vi "NodeFactory.vi"(8 "error in":errorcluster, 11 "reference":refnum<vi>) -> (0 "error out":errorcluster, 3 "Node out":refnum<class "Node.lvclass">)   [LabVIEW 2014, in "Raspberry Pi Compatible Compiler for LabVIEW.lvlib" / "Node.lvclass"]
uses:
  Node.lvclass
  Function/Function.lvclass
  Structure/Structure.lvclass
  GrowableFunction/GrowableFunction.lvclass
  SubVI/SubVI.lvclass
  Local/Local.lvclass
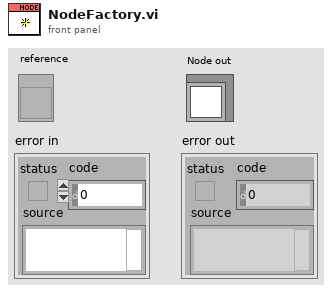
[diagram p1: front panel]
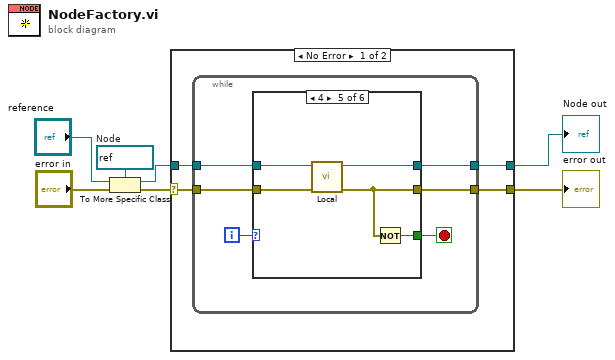
[diagram p0: block diagram]
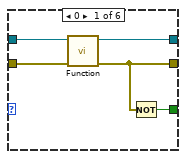
[diagram p2: hidden frame]
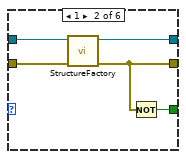
[diagram p3: hidden frame]
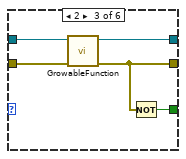
[diagram p4: hidden frame]
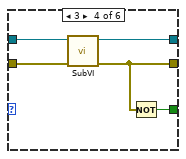
[diagram p5: hidden frame]
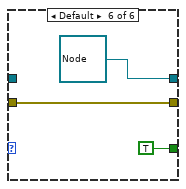
[diagram p6: hidden frame]
diagram:
  w5 = refnum<vi> refnum  # Node
  n1 = To More Specific Class(target class=w5, reference="reference", error in="error in") -> (specific class reference=w2:refnum<vi>, error out=w3:errorcluster)
  n2 = case shown="No Error" w3 {
    selector: w3 -> [w11 w46]
    tunnel: [w9 _] -> w7
    tunnel: [w8 w46] -> w6
    tunnel: w2 -> [w10 _]
    frame No Error {
      n3 = while {
        tunnel: w11 -> [w16]
        tunnel: [w15] -> w8
        tunnel: [w14] -> w9
        tunnel: w10 -> [w12]
        i -> [w17]
        stop <- w13 stop-if-true
        n4 = case shown="4" w17 {
          tunnel: w16 -> [w22 w27 w32 w37 w42 w44]
          tunnel: [w19 w24 w29 w34 w39 w44] -> w15
          tunnel: [w21 w26 w31 w36 w41 refnum<class "Node.lvclass"> refnum ("Node out")] -> w14
          tunnel: [w20 w25 w30 w35 w40 TRUE] -> w13
          tunnel: w12 -> [w18 w23 w28 w33 w38 _]
          frame 0 {
            n5 = call "Function.vi"("error in"=w22, "reference"=w18) -> ("error out"=w19:errorcluster, "Function out"=w21:refnum<class "Function.lvclass">)  [unwired: 8 in]
            n6 = Not(x=w19) -> (.not. x?=w20:bool)
          }
          frame 1 {
            n7 = call "StructureFactory.vi"("error in"=w27, "reference"=w23) -> ("error out"=w24:errorcluster, "structure out"=w26:refnum<class "Structure.lvclass">)  [unwired: 8 in]
            n8 = Not(x=w24) -> (.not. x?=w25:bool)
          }
          frame 2 {
            n9 = call "GrowableFunction.vi"("error in"=w32, "reference"=w28) -> ("error out"=w29:errorcluster, "Function out"=w31:refnum<class "GrowableFunction.lvclass">)  [unwired: 8 in]
            n10 = Not(x=w29) -> (.not. x?=w30:bool)
          }
          frame 3 {
            n11 = call "SubVI.vi"("error in"=w37, "reference"=w33) -> ("error out"=w34:errorcluster, "SubVI out"=w36:refnum<class "SubVI.lvclass">)  [unwired: 8 in]
            n12 = Not(x=w34) -> (.not. x?=w35:bool)
          }
          frame 4 {
            n13 = call "Local.vi"("error in"=w42, "reference"=w38) -> ("error out"=w39:errorcluster, "Local out"=w41:refnum<class "Local.lvclass">)  [unwired: 8 in]
            n14 = Not(x=w39) -> (.not. x?=w40:bool)
          }
          frame Default {
          }
        }
      }
    }
    frame Error {
    }
  }
  "error out" <- w6
  "Node out" <- w7
